vi "mainActivity__viOpen.vi"(8 "error in":errorcluster, 10 "subPane":refnum<vi>, 11 "数组":string[](array[string])) -> (0 "error out":errorcluster, 3 "viPath":path)   [LabVIEW 2014]
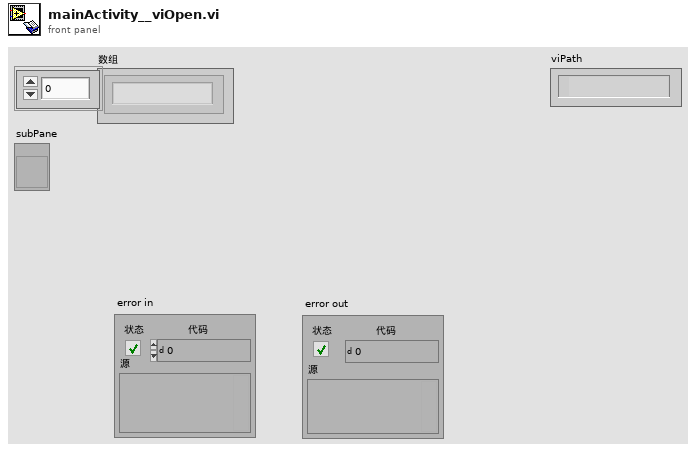
[diagram p1: front panel]
types:
  T1 = enum32{"Invalid", "Standard", "Closed", "Hidden", "Minimized", "Maximized"}
  T2 = enum32{"Bad", "Idle", "Run top level", "Running"}
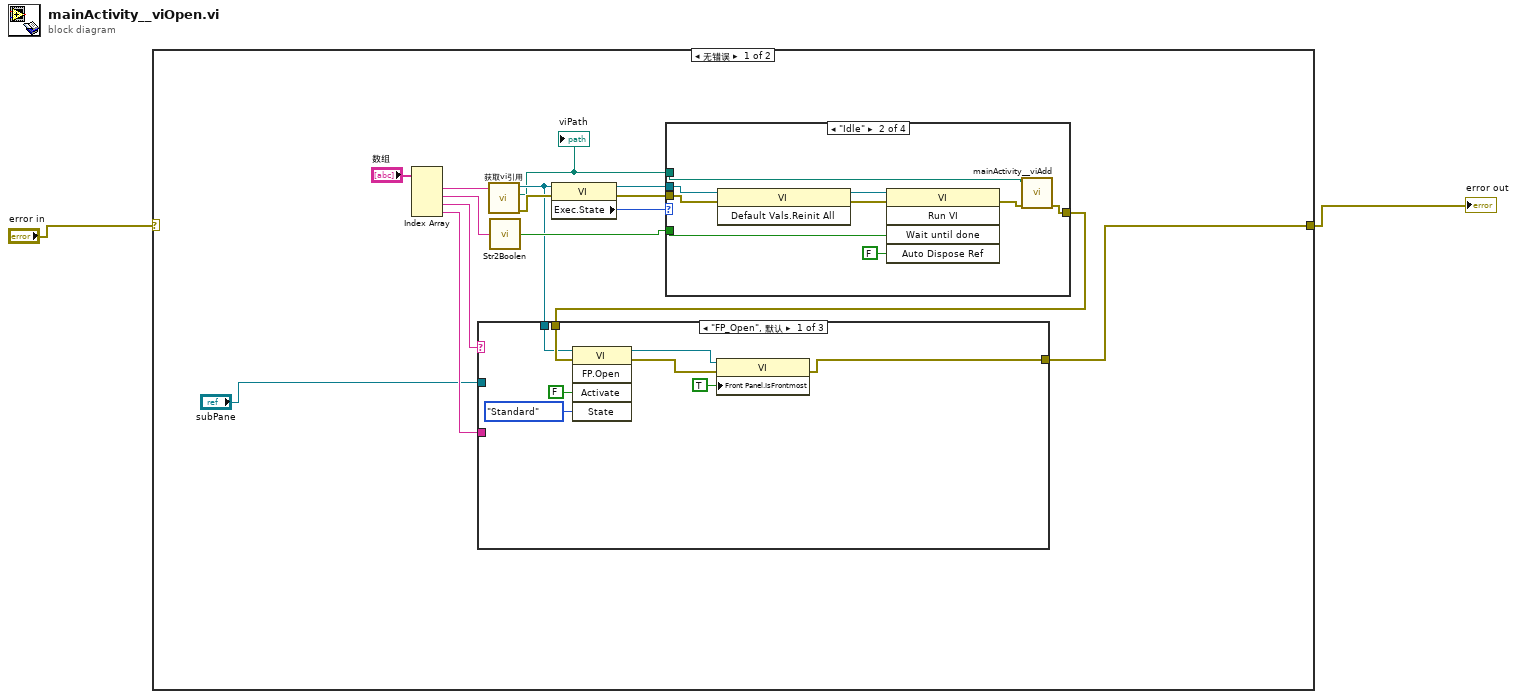
[diagram p0: block diagram]
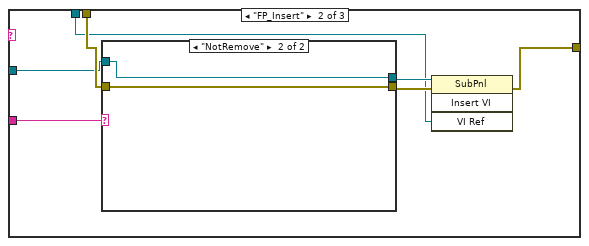
[diagram p2: hidden frame]
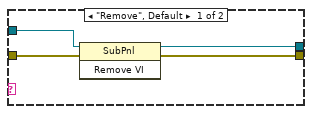
[diagram p3: hidden frame]
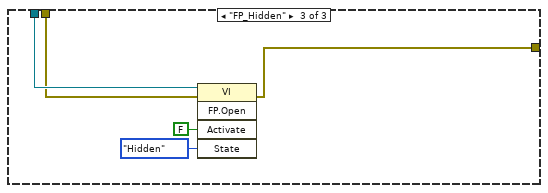
[diagram p4: hidden frame]
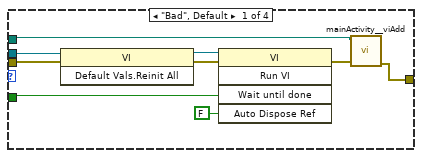
[diagram p5: hidden frame]
diagram:
  n1 = case shown="无错误" "error in" {
    selector: "error in" -> [_ w64]
    tunnel: [w5 w64] -> w1
    frame No Error {
      n2 = Index Array(array="数组") -> (element #1=w17:string, element #2=w12:string, element #3=w10:string, element #4=w7:string)  [unwired: 4 in]
      n3 = call "获取vi引用.vi"("urlStr"=w17) -> ("error out"=w16:errorcluster, "viPath"=w3:path, "VIOut"=w9:refnum<vi>)  [unwired: 8 in]
      "viPath" <- w3
      n4 = call "Str2Boolen.vi"("Str"=w12) -> ("Boolen"=w11:bool)
      n5 = property class="VI"(reference=w9, error in=w16) -> (reference out=w14:refnum<vi>, error out=w13:errorcluster, "Exec.State"=w15:T2)
      n6 = case shown="\"Idle\"" w15 {
        tunnel: w14 -> [w50 w59 _ _]
        tunnel: w13 -> [w47 w58 w62 w63]
        tunnel: w11 -> [w52 w61 _ _]
        tunnel: [w44 w54 w62 w63] -> w8
        tunnel: w3 -> [w46 w55 _ _]
        frame "Bad", Default {
          n7 = invoke class="VI" method="Default Vals.Reinit All"(reference=w50, error in=w47) -> (reference out=w49:refnum<vi>, error out=w48:errorcluster)  [unwired: 1 in, 1 out]
          n8 = invoke class="VI" method="Run VI"(reference=w49, error in=w48, "Wait until done"=w52, "Auto Dispose Ref"=FALSE ("自动销毁引用")) -> (error out=w45:errorcluster)  [unwired: 1 in, 4 out]
          n9 = call "mainActivity__viAdd.vi"("error in"=w45, "VI"=w46) -> ("error out"=w44:errorcluster)  [unwired: 9 in]
        }
        frame "Idle" {
          n10 = invoke class="VI" method="Default Vals.Reinit All"(reference=w59, error in=w58) -> (reference out=w56:refnum<vi>, error out=w57:errorcluster)  [unwired: 1 in, 1 out]
          n11 = invoke class="VI" method="Run VI"(reference=w56, error in=w57, "Wait until done"=w61, "Auto Dispose Ref"=FALSE ("自动销毁引用")) -> (error out=w53:errorcluster)  [unwired: 1 in, 4 out]
          n12 = call "mainActivity__viAdd.vi"("error in"=w53, "VI"=w55) -> ("error out"=w54:errorcluster)  [unwired: 9 in]
        }
        frame "Run top level" {
        }
        frame "Running" {
        }
      }
      n13 = case shown="\"FP_Open\", 默认" w10 {
        tunnel: w9 -> [w24 w28 w43]
        tunnel: w8 -> [w25 w31 w42]
        tunnel: [w19 w27 w41] -> w5
        tunnel: w7 -> [_ w32 _]
        tunnel: "subPane" -> [_ w26 _]
        frame "FP_Open", Default {
          n14 = invoke class="VI" method="FP.Open"(reference=w24, error in=w25, "Activate"=FALSE ("激活？"), "State"=T1."Standard" ("状态")) -> (reference out=w21:refnum<vi>, error out=w20:errorcluster)  [unwired: 1 in, 3 out]
          n15 = property class="VI"(reference=w21, error in=w20, "Front Panel.IsFrontmost"=TRUE ("前面板窗口:在最前")) -> (error out=w19:errorcluster)  [unwired: 1 out]
        }
        frame "FP_Insert" {
          n16 = case shown="\"NotRemove\"" w32 {
            tunnel: w26 -> [w36 w38]
            tunnel: w31 -> [w35 w37]
            tunnel: [w34 w37] -> w29
            tunnel: [w33 w38] -> w30
            frame "Remove", Default {
              n17 = invoke class="SubPnl" method="Remove VI"(reference=w36, error in=w35) -> (reference out=w33:refnum<vi>, error out=w34:errorcluster)  [unwired: 1 in, 1 out]
            }
            frame "NotRemove" {
            }
          }
          n18 = invoke class="SubPnl" method="Insert VI"(reference=w30, error in=w29, "VI Ref"=w28) -> (error out=w27:errorcluster)  [unwired: 1 in, 3 out]
        }
        frame "FP_Hidden" {
          n19 = invoke class="VI" method="FP.Open"(reference=w43, error in=w42, "Activate"=FALSE ("激活？"), "State"=T1."Hidden" ("状态")) -> (error out=w41:errorcluster)  [unwired: 1 in, 4 out]
        }
      }
    }
    frame Error {
    }
  }
  "error out" <- w1
